vi "Main.vi"(10 "Acq. Panel":refnum<vi>, 11 "Module Admin":refnum<class "Delacor_lib_QMH_Module Admin.lvclass">) -> ()   [LabVIEW 2020, in "Acquisition.lvlib"]
doc: "This template is based off of the Queued Message Handler design pattern and the Queued Message Handler project template that ships with LabVIEW.\n\nThe main difference is that the queue is private to this module and communication between modules is performed via Broadcast and Request events.\n\nRequest events are wrapped in public API methods and are handled in the Event Handling Loop (EHL) of this VI. Any module can register for Broadcast events sent by this module. The EHL generates messages based on user interface actions.\n\nThe Message Handling Loop (MHL) processes messages generated by the EHL, or by other messages. The messages are string values, so new messages can be added easily to the Message Cases case structure in the MHL. Each message cluster can also provide an optional value for Message Data, which is a variant that can be converted to whatever message-specific data is required.\n_____\nBased on Delacor QMH Project Template 5.0.0.82."
uses:
  Acquisition.lvlib
  <vilib>/Delacor/Delacor QMH/Libraries/Module Admin_class/Delacor_lib_QMH_Module Admin.lvclass
  Module Data--cluster.ctl
  <vilib>/Delacor/Delacor QMH/Libraries/Message Queue_class/Delacor_lib_QMH_Message Queue.lvclass/Delacor_lib_QMH_Message Queue.ctl
  Stop Argument--cluster.ctl
  <vilib>/Delacor/Delacor QMH/Libraries/Module Admin_class/Delacor_lib_QMH_Module Admin.lvclass/Delacor_lib_QMH_Module Admin.ctl
  Start ACQ Argument--cluster.ctl
  Stop Acq Argument--cluster.ctl
  <vilib>/Utility/miscctls.llb/LVPointTypeDef.ctl
  <vilib>/Delacor/Delacor QMH/Libraries/Message Queue_class/Delacor_lib_QMH_Enqueue Message (Single).vi
  <vilib>/Delacor/Delacor QMH/Libraries/Module Admin_class/Delacor_lib_QMH_Get External Launch.vi
  <vilib>/Utility/error.llb/Error Cluster From Error Code.vi
  <vilib>/ErrorRing/Error Ring.xnode
  <vilib>/Delacor/Delacor QMH/Libraries/Message Queue_class/Delacor_lib_QMH_Message Queue.lvclass
  <vilib>/measure/NI_MABase.lvlib
panel:
  out "Waveform Graph":waveform(dbl)(graph)
  in  "Simulate MHL Error":bool
  in  "Simulate EHL Error":bool
  out "error out":errorcluster
  out "Status":string
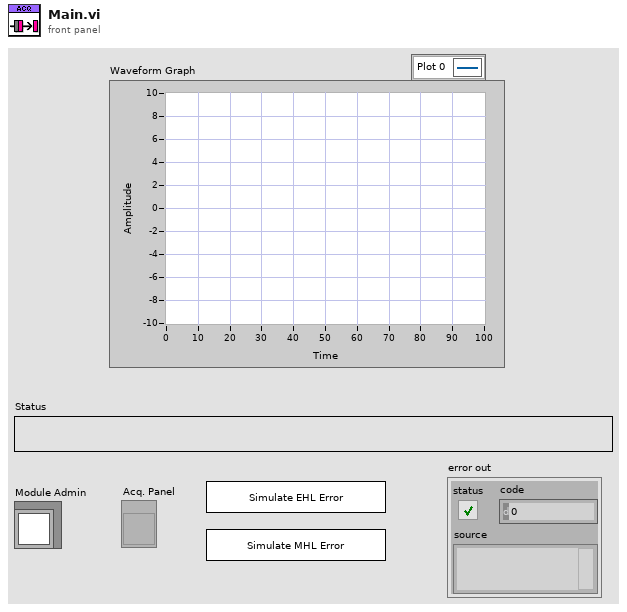
[diagram p1: front panel]
types:
  T1 = typedef "Acquisition.lvlib/Request Events--cluster.ctl" = cluster{"Stop Module":refnum<user-event>, "Show Panel":refnum<user-event>, "Hide Panel":refnum<user-event>, "Get Module Execution Status":refnum<user-event>, "Show Diagram":refnum<user-event>, "Start ACQ":refnum<user-event>, "Stop Acq":refnum<user-event>}
  T2 = typedef "Acquisition.lvlib/Module Data--cluster.ctl" = cluster{"Status":string}
  T3 = enum32{"invalid lock state", "Not Locked", "Locked (No Password)", "Password-protected"}
  T4 = typedef "Acquisition.lvlib/Stop Argument--cluster.ctl" = cluster{"Origin":string, "Exit via Stop Module Req?":bool, "Wait for Module to stop?":bool}
  T5 = typedef "Acquisition.lvlib/Start ACQ Argument--cluster.ctl" = cluster{"Boolean":bool}
  T6 = typedef "Acquisition.lvlib/Stop Acq Argument--cluster.ctl" = cluster{"Boolean":bool}
  T7 = typedef "LVPointTypeDef.ctl" = cluster{"Horizontal":i16, "Vertical":i16}
  T8 = enum32{"Invalid", "Standard", "Closed", "Hidden", "Minimized", "Maximized"}
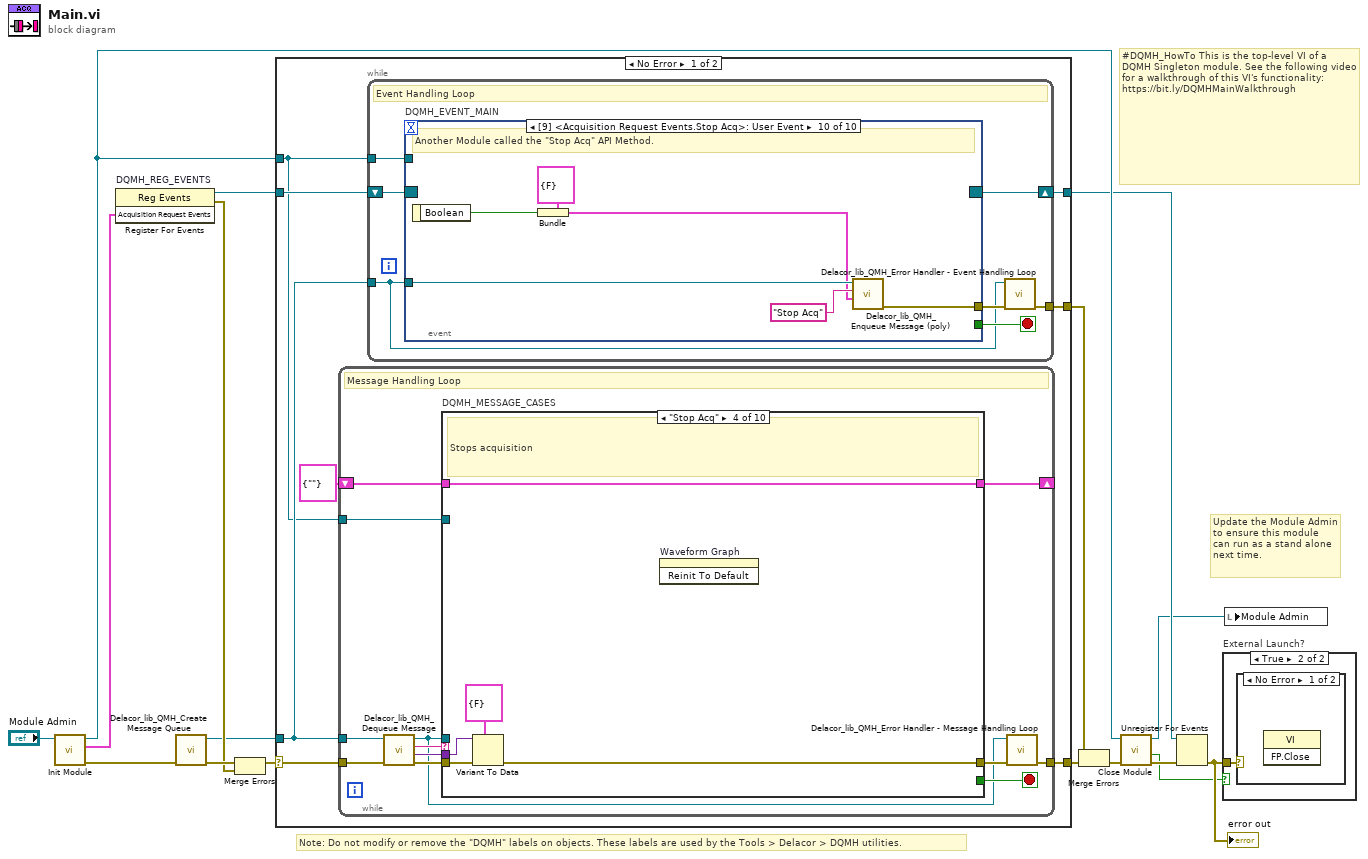
[diagram p0: block diagram]
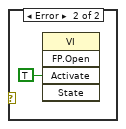
[diagram p3: hidden frame]
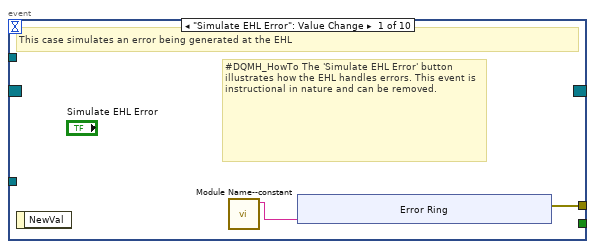
[diagram p4: hidden frame]
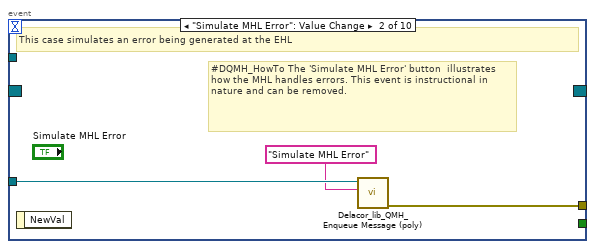
[diagram p5: hidden frame]
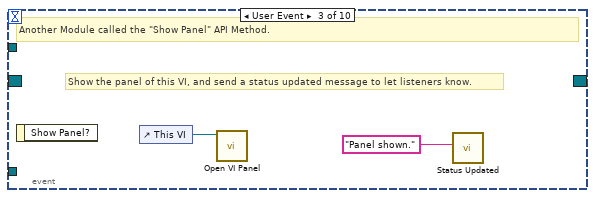
[diagram p6: hidden frame]
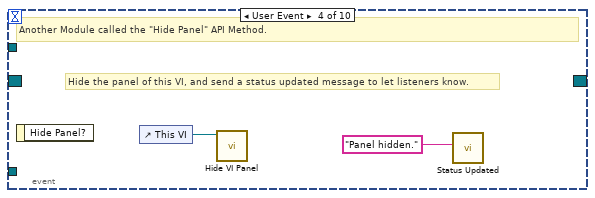
[diagram p7: hidden frame]
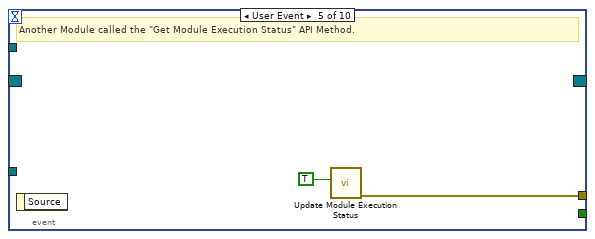
[diagram p8: hidden frame]
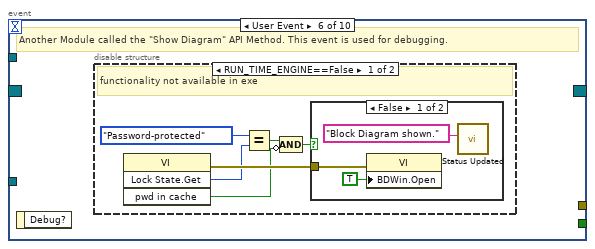
[diagram p9: hidden frame]
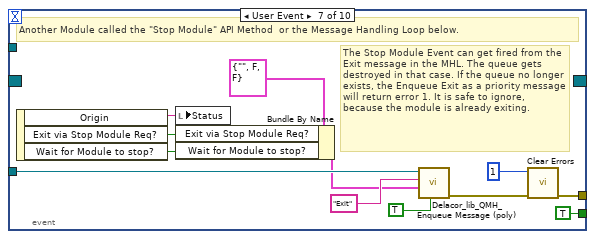
[diagram p12: hidden frame]
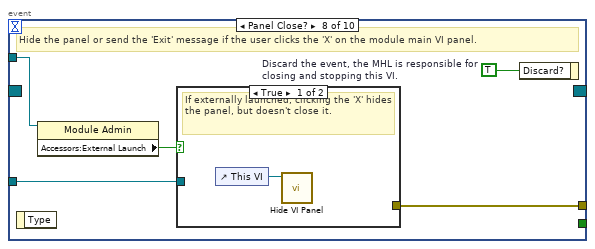
[diagram p13: hidden frame]
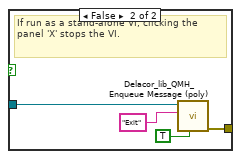
[diagram p14: hidden frame]
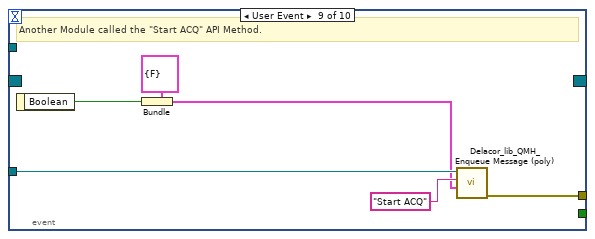
[diagram p15: hidden frame]
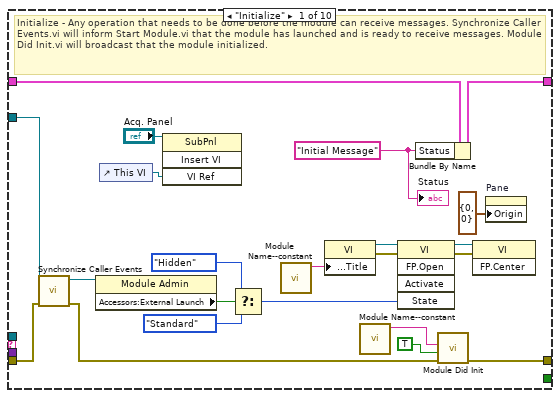
[diagram p16: hidden frame]
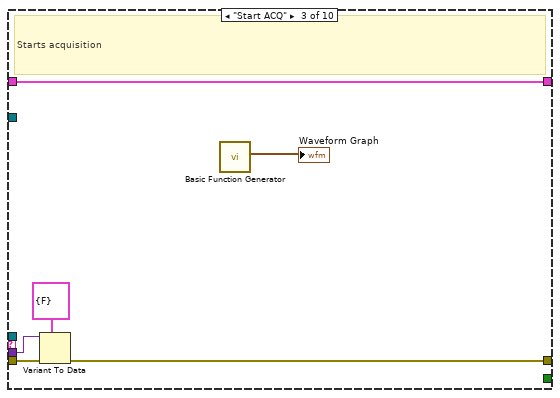
[diagram p18: hidden frame]
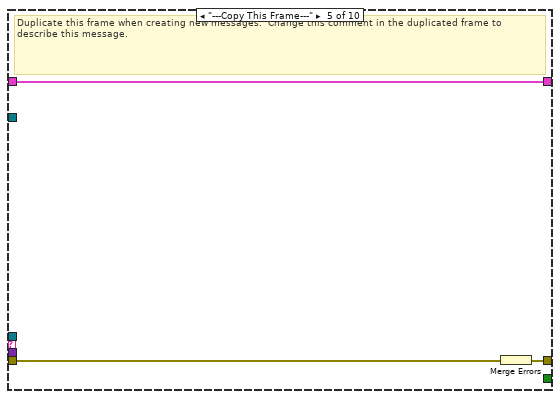
[diagram p19: hidden frame]
diagram:
  # "#DQMH_HowTo This is the top-level VI of a DQMH Singleton module. See the following video for a walkthrough of this VI's functionality: https://bit.ly/DQMHMainWalkthrough"
  # "Note: Do not modify or remove the \"DQMH\" labels on objects. These labels are used by the Tools > Delacor > DQMH utilities."
  # "Update the Module Admin to ensure this module can run as a stand alone next time."
  n1 = call "Init Module.vi"("Singleton Module Admin in"="Module Admin") -> ("error out"=w16:errorcluster, "Acquisition Request Events"=w5:T1, "Singleton Module Admin out"=w8:refnum<class "Delacor_lib_QMH_Module Admin.lvclass">)  [unwired: 8 in]
  n2 = register-events "DQMH_REG_EVENTS"(w5) -> (reference out=w6:refnum<event-registration>, error out=w9:errorcluster)  [unwired: 2 in]
  n3 = call <vilib>:"Delacor_lib_QMH_Create Message Queue.vi"("error in (no error)"=w16) -> ("error out"=w11:errorcluster, "Message Queue"=w4:refnum<class "Delacor_lib_QMH_Message Queue.lvclass">)  [unwired: 9 in]
  n4 = Merge Errors(w11, w9) -> (w10:errorcluster)
  n5 = case shown="No Error" w10 {
    selector: w10 -> [w23 w206]
    tunnel: [w25 w205] -> w17
    tunnel: [w22 w211] -> w7
    tunnel: w6 -> [w20 w211]
    tunnel: w4 -> [w19 w204]
    tunnel: [w24 _] -> w14
    tunnel: w8 -> [w18 w207]
    frame No Error {
      n6 = while {
        tunnel: w19 -> [w96]
        shift-right: [w100] -> _
        shift-left: T2 {"Status"=""} ("Data Cluster") -> [w101]
        tunnel: w23 -> [w104]
        tunnel: [w102] -> w25
        tunnel: w18 -> [w94]
        stop <- w99 stop-if-true
        # "Message Handling Loop"
        n7 = call-dynamic "Delacor_lib_QMH_Dequeue Message.vi"("error in (no error)"=w104, "Message Queue in"=w96) -> ("error out"=w103:errorcluster, "Message Data"=w97:variant, "Message"=w98:string, "Message Queue out"=w95:refnum<class "Delacor_lib_QMH_Message Queue.lvclass">)  [unwired: 6 in]
        n8 = case "DQMH_MESSAGE_CASES" shown="\"Stop Acq\"" w98 {
          selector: w98 -> [_ _ _ _ _ _ _ _ _ w191]
          tunnel: w95 -> [_ _ _ _ _ _ _ w161 w183 _]
          tunnel: w103 -> [w125 w129 w135 w140 w143 w145 w150 w168 w189 w193]
          tunnel: [w123 w129 w133 w138 w142 w145 w149 w164 w186 w194] -> w105
          tunnel: w101 -> [w114 w128 w134 w139 w141 w144 w147 w163 w182 w192]
          tunnel: [w113 w128 w134 w139 w141 w144 w147 w163 w182 w192] -> w100
          tunnel: [_ _ _ _ _ _ _ _ w181 _] -> w99
          tunnel: w97 -> [_ _ w132 w137 _ _ _ w162 w180 _]
          tunnel: w94 -> [w115 _ _ _ _ _ _ w160 w175 _]
          frame "Initialize" {
            w108 = "Initial Message" ("Initial Message")
            # "Initialize - Any operation that needs to be done before the module can receive messages. Synchronize Caller Events.vi will inform Start Module.vi that the module has launched and is ready to receive messages. Module Did Init.vi will broadcast that the module initialized."
            n9 = call "Synchronize Caller Events.vi"("error in (no error)"=w125, "Singleton Module Admin in"=w115) -> ("error out"=w124:errorcluster, "Singleton Module Admin out"=w110:refnum<class "Delacor_lib_QMH_Module Admin.lvclass">)  [unwired: 8 in]
            n10 = property class="Module Admin"(reference=w110) -> ("Accessors:External Launch"=w119:bool)  [unwired: 1 in, 2 out]
            n11 = control-ref of="This VI"() -> (w106:refnum<vi>)
            n12 = invoke class="SubPnl" method="Insert VI"(reference="Acq. Panel", "VI Ref"=w106) -> ()  [unwired: 2 in, 4 out]
            n13 = Select(t=T8."Hidden" ("State"), s=w119, f=T8."Standard" ("State")) -> (s? t:f=w116:T8)
            n14 = call "Module Name--constant.vi"() -> ("Module Name"=w122:string)  [unwired: 11 in]
            n15 = property class="VI"("Front Panel.Title"=w122) -> (reference out=w121:refnum<vi>, error out=w127:errorcluster)  [unwired: 2 in]
            n16 = call "Module Name--constant.vi"() -> ("Module Name"=w111:string)  [unwired: 11 in]
            n17 = invoke class="VI" method="FP.Open"(reference=w121, error in=w127, "State"=w116) -> (reference out=w120:refnum<vi>, error out=w126:errorcluster)  [unwired: 2 in, 3 out]
            n18 = Bundle By Name(cluster=w114, "Status"=w108) -> (w113:T2)
            n19 = call "Module Did Init.vi"("error in (no error)"=w124, "Initialized?"=TRUE, "Origin"=w111) -> ("error out"=w123:errorcluster)  [unwired: 8 in]
            n20 = invoke class="VI" method="FP.Center"(reference=w120, error in=w126) -> ()  [unwired: 1 in, 3 out]
            n21 = property on="Pane" class="Pane"("Origin"=T7 {"Horizontal"=0, "Vertical"=0}) -> ()  [unwired: 2 in, 2 out]
            "Status" <- w108
          }
          frame "--- Module Specific ---" {
            # "Separator -- The following cases handle messages specific to this Module."
          }
          frame "Start ACQ" {
            # "Starts acquisition"
            n22 = Variant To Data(error in=w135, type=T5 {"Boolean"=FALSE} ("Start ACQ Argument"), Variant=w132) -> (error out=w133:errorcluster)  [unwired: 1 out]
            n23 = call <vilib>:"Basic Function Generator.vi"() -> ("signal out"=→"Waveform Graph":waveform(dbl))  [unwired: 9 in, 2 out]
          }
          frame "Stop Acq" {
            # "Stops acquisition"
            n24 = Variant To Data(error in=w140, type=T6 {"Boolean"=FALSE} ("Stop Acq Argument"), Variant=w137) -> (error out=w138:errorcluster)  [unwired: 1 out]
            n25 = invoke on="Waveform Graph" class="WFGraph (strict)" method="Reinit To Default"() -> ()  [unwired: 3 in, 3 out]
          }
          frame "---Copy This Frame---" {
            # "Duplicate this frame when creating new messages.  Change this comment in the duplicated frame to describe this message."
            n26 = Merge Errors(w143) -> (w142:errorcluster)
          }
          frame "--- Exit and Error Handling---" {
            # "Separator - The following cases handle errors and exit messages."
          }
          frame "Simulate MHL Error" {
            # "#DQMH_HowTo The 'Simulate MHL Error' button  illustrates how the MHL handles errors. This event is instructional in nature and can be removed."
            # "Simulate an error occurring at the MHL"
            n27 = call "Module Name--constant.vi"() -> ("Module Name"=w146:string)  [unwired: 11 in]
            n28 = xnode "Error Ring"("parameter 0"=w146) -> ("error out"=w148:errorcluster)
            n29 = Merge Errors(w150, w148) -> (w149:errorcluster)
          }
          frame "Error" {
            # "#CodeRecommended - If you ever change the name of this \"Error\" message, you'll need to update the name in the Check Loop Error.vi as well."
            # "#CodeRecommended - If the module is running in standalone mode (External Launch = FALSE), this code will pop up an error dialog and call the 'Exit' message if an error occurs. Add more fine-grained error handling here."
            # "Error - Check the error message data and respond accordingly. This message is sent by the \"Error Handler\" VIs at the end of each loop in this application."
            n30 = property class="Module Admin"(reference=w160) -> ("Accessors:External Launch"=w159:bool)  [unwired: 1 in, 2 out]
            n31 = Variant To Data(error in=w168, type=errorcluster {"status"=FALSE, "code"=0, "source"=""} ("error constant"), Variant=w162) -> (data=w169:errorcluster, error out=w166:errorcluster)
            n32 = call "Module Name--constant.vi"() -> ("Module Name"=w158:string)  [unwired: 11 in]
            n33 = call "Error Reported.vi"("Additional Information"=w158, "Error"=w169) -> ()  [unwired: 9 in, 1 out]
            n34 = case shown="False" w159 {
              tunnel: [w174 _] -> w165
              tunnel: w161 -> [w172 _]
              tunnel: w169 -> [w173 _]
              frame False {
                # "If the module is running standalone, then pop up an error dialog and call the \"Exit\" message."
                n35 = call <vilib>:"Simple Error Handler.vi"("error in (no error)"=w173) -> ()  [unwired: 4 in, 5 out]
                n36 = call-poly <vilib>:"Delacor_lib_QMH_Enqueue Message (poly).vi"("Priority Message? (F)"=TRUE, "Message"="Exit", "Message Queue in"=w172) -> ("error out"=w174:errorcluster)  [unwired: 7 in, 1 out]
              }
              frame True {
                # "If the module was launched externally, calling the Error Reported broadcast VI is the only action performed by the \"Error\" message. The module's caller can then process the error appropriately."
              }
            }
            n37 = Merge Errors(w166, w165) -> (w164:errorcluster)
            n38 = local write "error out"(w164) -> ()
          }
          frame "Exit" {
            w179 = 91  # 91: not all Exit messages will have an argument
            w181 = TRUE  # Stop the VI
            # "Release the message queue reference"
            # "#CodeNeeded - Add any required cleanup code here"
            # "Exit - Exit the application."
            n39 = Variant To Data(error in=w189, type=T4 {"Origin"="", "Exit via Stop Module Req?"=FALSE, "Wait for Module to stop?"=FALSE} ("Stop Argument"), Variant=w180) -> (data=w177:T4, error out=w185:errorcluster)
            n40 = call <vilib>:"Clear Errors.vi"("error in (no error)"=w185, "specific error code to clear (0: all)"=w179) -> ("error out"=w188:errorcluster)  [unwired: 4 in, 1 out]
            n41 = control-ref of="This VI"() -> (w176:refnum<vi>)
            n42 = call-dynamic "Delacor_lib_QMH_Release Message Queue.vi"("error in (no error)"=w188, "Message Queue"=w183) -> ("error out"=w187:errorcluster)  [unwired: 9 in]
            n43 = call "Handle Exit.vi"("Stop Argument"=w177, "Admin in"=w175, "VI reference"=w176) -> ("error out"=w184:errorcluster)  [unwired: 7 in, 1 out]
            n44 = Merge Errors(w187, w184) -> (w186:errorcluster)
          }
          frame Default {
            # "'Default' case only runs if there is a message that isn't defined in any of the other cases.  Output a programming error."
            n45 = call "Module Name--constant.vi"() -> ("Module Name"=w190:string)  [unwired: 11 in]
            n46 = xnode "Error Ring"("parameter 0"=w191, "parameter 1"=w190) -> ("error out"=w195:errorcluster)
            n47 = Merge Errors(w193, w195) -> (w194:errorcluster)
          }
        }
        n48 = call-dynamic "Delacor_lib_QMH_Error Handler - Message Handling Loop.vi"("error in (no error)"=w105, "Message Queue in"=w95) -> ("dup error in"=w102:errorcluster)  [unwired: 8 in, 1 out]
      }
      n49 = while {
        tunnel: w19 -> [w26]
        shift-right: [w29] -> w22
        shift-left: w20 -> [w30]
        tunnel: [w31] -> w24
        tunnel: w18 -> [w27]
        stop <- w28 stop-if-true
        # "Event Handling Loop"
        n50 = event "DQMH_EVENT_MAIN" shown="[9] <Acquisition Request Events.Stop Acq>: User Event" {
          selector: w30 -> [_ _ _ _ _ _ _ _ _ _]
          dyn-events: [_ _ _ _ _ _ _ _ _ _] -> w29
          timeout: _ -> [_ _ _ _ _ _ _ _ _ _]
          tunnel: [_ _ _ _ _ _ TRUE ("Discard?") _ _ _] -> w28
          tunnel: w26 -> [_ w43 _ _ _ _ w67 w74 w87 w93]
          tunnel: [w34 w44 _ _ w50 _ w70 w76 w82 w88] -> w32
          tunnel: w27 -> [_ _ _ _ _ _ _ w73 _ _]
          event "Simulate EHL Error": Value Change {
            # "#DQMH_HowTo The 'Simulate EHL Error' button  illustrates how the EHL handles errors. This event is instructional in nature and can be removed."
            # "This case simulates an error being generated at the EHL"
            n51 = event-data() -> ()  [unwired: 1 in, 1 out]
            n52 = call "Module Name--constant.vi"() -> ("Module Name"=w33:string)  [unwired: 11 in]
            n53 = xnode "Error Ring"("parameter 0"=w33) -> ("error out"=w34:errorcluster)
          }
          event "Simulate MHL Error": Value Change {
            # "#DQMH_HowTo The 'Simulate MHL Error' button  illustrates how the MHL handles errors. This event is instructional in nature and can be removed."
            # "This case simulates an error being generated at the EHL"
            n54 = event-data() -> ()  [unwired: 1 in, 1 out]
            n55 = call-poly <vilib>:"Delacor_lib_QMH_Enqueue Message (poly).vi"("Message"="Simulate MHL Error", "Message Queue in"=w43) -> ("error out"=w44:errorcluster)  [unwired: 8 in, 1 out]
          }
          event User Event {
            # "Show the panel of this VI, and send a status updated message to let listeners know."
            # "Another Module called the \"Show Panel\" API Method."
            n56 = event-data() -> ()  [unwired: 1 in, 1 out]
            n57 = control-ref of="This VI"() -> (w46:refnum<vi>)
            n58 = call "Open VI Panel.vi"("VI"=w46) -> ()  [unwired: 10 in, 1 out]
            n59 = call "Status Updated.vi"("Status"="Panel shown." ("format string")) -> ()  [unwired: 10 in, 1 out]
          }
          event User Event {
            # "Hide the panel of this VI, and send a status updated message to let listeners know."
            # "Another Module called the \"Hide Panel\" API Method."
            n60 = event-data() -> ()  [unwired: 1 in, 1 out]
            n61 = control-ref of="This VI"() -> (w48:refnum<vi>)
            n62 = call "Hide VI Panel.vi"("VI"=w48) -> ()  [unwired: 10 in, 1 out]
            n63 = call "Status Updated.vi"("Status"="Panel hidden." ("format string")) -> ()  [unwired: 10 in, 1 out]
          }
          event User Event {
            # "Another Module called the \"Get Module Execution Status\" API Method."
            n64 = event-data() -> ()  [unwired: 1 in, 1 out]
            n65 = call "Update Module Execution Status.vi"("Running?"=TRUE) -> ("error out"=w50:errorcluster)  [unwired: 10 in]
          }
          event User Event {
            # "Another Module called the \"Show Diagram\" API Method. This event is used for debugging."
            n66 = event-data() -> ()  [unwired: 1 in, 1 out]
            n67 = disable-structure shown="RUN_TIME_ENGINE==False" {
              frame condition #0 (active) {
                # "functionality not available in exe"
                n68 = invoke class="VI" method="Lock State.Get"() -> (error out=w56:errorcluster, "Get Lock State"=w55:T3, "pwd in cache"=w52:bool)  [unwired: 4 in, 1 out]
                n69 = Equal?(x=T3."Password-protected", y=w55) -> (x = y?=w53:bool)
                n70 = Compound Arithmetic op=AND(w53, invert w52) -> (w51:bool)
                n71 = case shown="False" w51 {
                  tunnel: w56 -> [w59 _]
                  frame False {
                    n72 = property class="VI"(error in=w59, "BDWin.Open"=TRUE ("Block Diagram Window:Open")) -> ()  [unwired: 1 in, 2 out]
                    n73 = call "Status Updated.vi"("Status"="Block Diagram shown." ("format string")) -> ()  [unwired: 10 in, 1 out]
                  }
                  frame True {
                    # "Password-protected VI, and the password is not in the cache. Do not show the diagram."
                  }
                }
              }
              frame condition #1 {
              }
            }
          }
          event User Event {
            # "The Stop Module Event can get fired from the Exit message in the MHL. The queue gets destroyed in that case. If the queue no longer exists, the Enqueue Exit as a priority message will return error 1. It is safe to ignore, because the module is already exiting."
            # "Another Module called the \"Stop Module\" API Method  or the Message Handling Loop below."
            n74 = event-data() -> ("Origin"=w66:string, "Exit via Stop Module Req?"=w62:bool, "Wait for Module to stop?"=w61:bool)  [unwired: 1 in]
            n75 = local write "Status"(w66) -> ()
            n76 = Bundle By Name(cluster=T4 {"Origin"="", "Exit via Stop Module Req?"=FALSE, "Wait for Module to stop?"=FALSE} ("Stop Argument"), "Exit via Stop Module Req?"=w62, "Wait for Module to stop?"=w61) -> (w60:T4)
            n77 = call-poly <vilib>:"Delacor_lib_QMH_Enqueue Message (poly).vi"("Priority Message? (F)"=TRUE, "Message Data"=w60, "Message"="Exit", "Message Queue in"=w67) -> ("error out"=w71:errorcluster)  [unwired: 6 in, 1 out]
            n78 = call <vilib>:"Clear Errors.vi"("error in (no error)"=w71, "specific error code to clear (0: all)"=1) -> ("error out"=w70:errorcluster)  [unwired: 4 in, 1 out]
          }
          event Panel Close? {
            w75 = TRUE  # Discard the event, the MHL is responsible for closing and stopping this VI.
            # "Hide the panel or send the 'Exit' message if the user clicks the 'X' on the module main VI panel."
            n79 = event-data() -> ()  [unwired: 1 in, 1 out]
            n80 = property class="Module Admin"(reference=w73) -> ("Accessors:External Launch"=w72:bool)  [unwired: 1 in, 2 out]
            n81 = case shown="True" w72 {
              tunnel: w74 -> [_ w80]
              tunnel: [_ w81] -> w76
              frame True {
                # "If externally launched, clicking the 'X' hides the panel, but doesn't close it."
                n82 = control-ref of="This VI"() -> (w77:refnum<vi>)
                n83 = call "Hide VI Panel.vi"("VI"=w77) -> ()  [unwired: 10 in, 1 out]
              }
              frame False {
                # "If run as a stand-alone VI, clicking the panel 'X' stops the VI."
                n84 = call-poly <vilib>:"Delacor_lib_QMH_Enqueue Message (poly).vi"("Priority Message? (F)"=TRUE, "Message"="Exit", "Message Queue in"=w80) -> ("error out"=w81:errorcluster)  [unwired: 7 in, 1 out]
              }
            }
            n85 = event-data("Discard?"=w75) -> ()  [unwired: 1 in, 1 out]
          }
          event User Event {
            # "Another Module called the \"Start ACQ\" API Method."
            n86 = event-data() -> ("Boolean"=w83:bool)  [unwired: 1 in]
            n87 = Bundle(cluster=T5 {"Boolean"=FALSE} ("Start ACQ Argument"), "Boolean"=w83) -> (w84:T5)
            n88 = call-poly <vilib>:"Delacor_lib_QMH_Enqueue Message (poly).vi"("Message Data"=w84, "Message"="Start ACQ", "Message Queue in"=w87) -> ("error out"=w82:errorcluster)  [unwired: 7 in, 1 out]
          }
          event User Event {
            # "Another Module called the \"Stop Acq\" API Method."
            n89 = event-data() -> ("Boolean"=w89:bool)  [unwired: 1 in]
            n90 = Bundle(cluster=T6 {"Boolean"=FALSE} ("Stop Acq Argument"), "Boolean"=w89) -> (w90:T6)
            n91 = call-poly <vilib>:"Delacor_lib_QMH_Enqueue Message (poly).vi"("Message Data"=w90, "Message"="Stop Acq", "Message Queue in"=w93) -> ("error out"=w88:errorcluster)  [unwired: 7 in, 1 out]
          }
        }
        n92 = call-dynamic "Delacor_lib_QMH_Error Handler - Event Handling Loop.vi"("error in (no error)"=w32, "Message Queue in"=w26) -> ("dup error in"=w31:errorcluster)  [unwired: 8 in, 1 out]
      }
    }
    frame Error {
      # "Synchronize Caller Events.vi will inform Start Module.vi that the module has launched and will let the code calling Start Module.vi register for broadcasts and would permit the caller receive the broadcast that an error occurred at launch time."
      n93 = call-dynamic "Delacor_lib_QMH_Release Message Queue.vi"("error in (no error)"=w206, "Message Queue"=w204) -> ("error out"=w205:errorcluster)  [unwired: 9 in]
      n94 = call "Synchronize Caller Events.vi"("Singleton Module Admin in"=w207) -> ("error out"=w212:errorcluster)  [unwired: 9 in, 1 out]
      n95 = call "Module Name--constant.vi"() -> ("Module Name"=w210:string)  [unwired: 11 in]
      n96 = Format Into String(format string="An error occurred during initialization. %s is no longer running.", w210) -> (resulting string=w208:string)  [unwired: 2 in, 1 out]
      n97 = Merge Errors(w205, w212) -> (w213:errorcluster)
      n98 = call "Error Reported.vi"("Additional Information"=w208, "Error"=w213) -> ()  [unwired: 9 in, 1 out]
    }
  }
  n99 = Merge Errors(w14, w17) -> (w13:errorcluster)
  n100 = call "Close Module.vi"("error in (no error)"=w13, "Module Admin in"=w8) -> ("error out"=w15:errorcluster, "External Launch"=w1:bool, "Module Admin out"=w2:refnum<class "Delacor_lib_QMH_Module Admin.lvclass">)  [unwired: 7 in]
  n101 = Unregister For Events(event registration refnum=w7, error in=w15) -> (error out=w12:errorcluster)
  "error out" <- w12
  n102 = case "External Launch?" shown="True" w1 {
    tunnel: w12 -> [_ w214]
    frame False {
    }
    frame True {
      n103 = case shown="No Error" w214 {
        frame No Error {
          n104 = invoke class="VI" method="FP.Close"() -> ()  [unwired: 3 in, 3 out]
        }
        frame Error {
          n105 = invoke class="VI" method="FP.Open"("Activate"=TRUE ("Activate?")) -> ()  [unwired: 4 in, 5 out]
        }
      }
    }
  }
  n106 = local write "Module Admin"(w2) -> ()
